vi "Twist3d_Create.vi"(4 "rZ":dbl, 6 "rY":dbl, 8 "rX":dbl, 9 "dZ":dbl, 10 "dY":dbl, 11 "dX":dbl) -> (3 "Twist3d":T1)   [LabVIEW 2019, in "Trajectory_Library.lvlib"]
doc: "Constructs a Twist3d with the given values.\n\n\nParameters:\n - dx - Change in x direction relative to robot.\n - dy - Change in y direction relative to robot.\n - dz - Change in z direction relative to robot.\n - rx - Rotation vector x component.\n - ry - Rotation vector y component.\n - rz - Rotation vector z component.\n\nResults:\n - TWIST3D - TWIST3D data structure"
uses:
  Trajectory_Library.lvlib
  TypeDef/TWIST3D.ctl
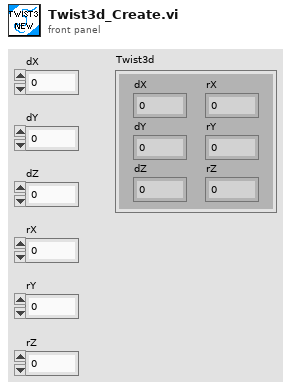
[diagram p1: front panel]
types:
  T1 = typedef "Trajectory_Library.lvlib/TWIST3D.ctl" = cluster{"dX":dbl, "dY":dbl, "dZ":dbl, "rX":dbl, "rY":dbl, "rZ":dbl}
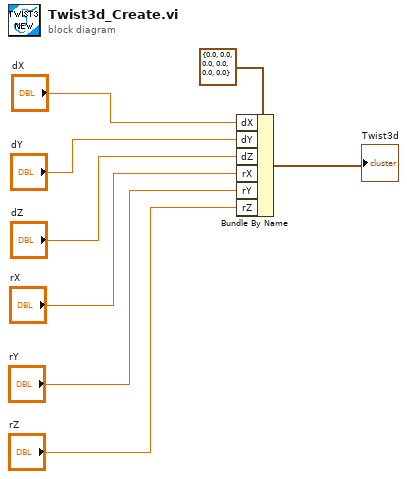
[diagram p0: block diagram]
diagram:
  n1 = Bundle By Name(cluster=T1 {"dX"=0.0, "dY"=0.0, "dZ"=0.0, "rX"=0.0, "rY"=0.0, "rZ"=0.0} ("TWIST"), "dX"="dX", "dY"="dY", "dZ"="dZ", "rX"="rX", "rY"="rY", "rZ"="rZ") -> (→"Twist3d":T1)
